vi "Automatische Umschaltung.vi"(6 "Aktion":T1, 8 "error in (no error)":errorcluster caption="Fehler (Eingang, kein Fehler)", 11 "TCP Connection":refnum<k5>) -> (0 "error out":errorcluster caption="Fehler (Ausgang)", 3 "TCP Connection":refnum<k5>)   [LabVIEW 2020, in "ABB-EL3000.lvlib" / "FID.lvlib"]
uses:
  FID.lvlib
  Aktion automatische Umschaltung.ctl
  FID Kalibrierung/Aktion FID Allgemeindaten.ctl
  Modus.ctl
  FID Kalibrierung/FID Kalibrierung.lvlib
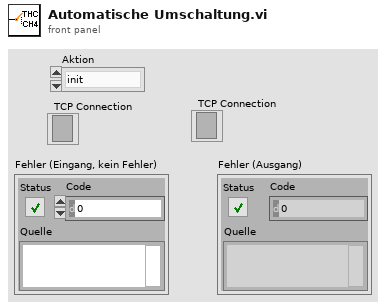
[diagram p1: front panel]
types:
  T1 = typedef "ABB-EL3000.lvlib/FID.lvlib/Aktion automatische Umschaltung.ctl" = enum16{"init", "lesen"}
  T2 = typedef "ABB-EL3000.lvlib/FID.lvlib/Modus.ctl" = enum16{"Automatic", "CH4", "THC", "Efficienty measure", "Switching time"}
  T3 = typedef "ABB-EL3000.lvlib/FID.lvlib/FID Kalibrierung.lvlib/Aktion FID Allgemeindaten.ctl" = enum16{"lesen", "Mod", "Time", "laden", "speichern"}
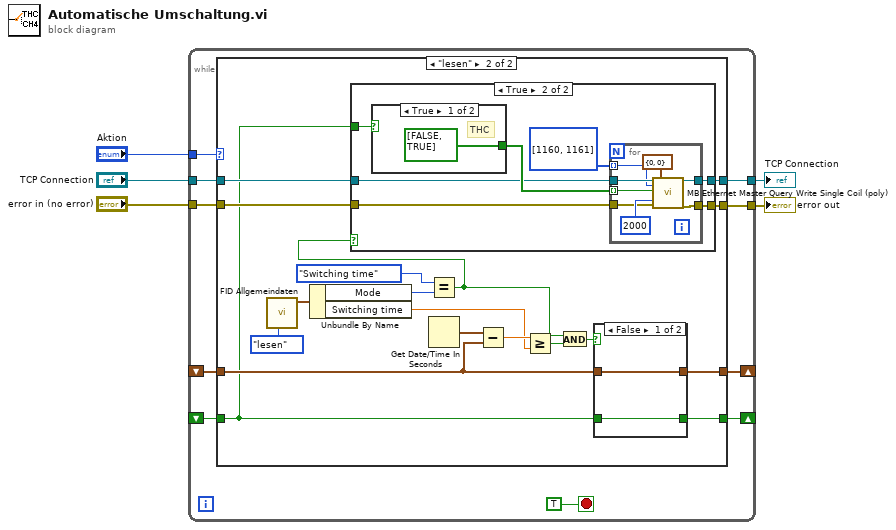
[diagram p0: block diagram]
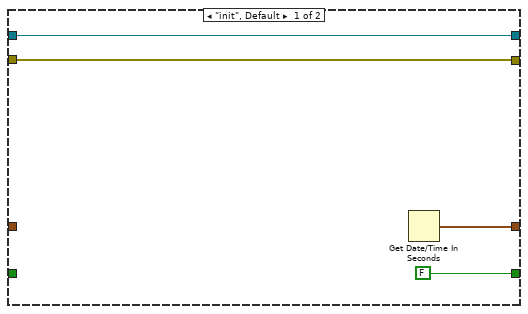
[diagram p2: hidden frame]
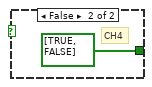
[diagram p4: hidden frame]
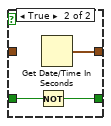
[diagram p5: hidden frame]
diagram:
  n1 = while {
    tunnel: "Aktion" -> [w14]
    shift-right: [w13] -> _
    shift-left: _ -> [w12]
    shift-right: [w11] -> _
    shift-left: _ -> [w10]
    tunnel: "error in (no error)" -> [w7]
    tunnel: "TCP Connection" -> [w9]
    tunnel: [w8] -> w3
    tunnel: [w6] -> w1
    stop <- TRUE stop-if-true
    n2 = case shown="\"lesen\"" w14 {
      tunnel: [w19 w32] -> w13
      tunnel: w12 -> [_ w33]
      tunnel: [FALSE w29] -> w11
      tunnel: w10 -> [_ w24]
      tunnel: w9 -> [w17 w28]
      tunnel: [w17 w27] -> w8
      tunnel: w7 -> [w16 w26]
      tunnel: [w16 w25] -> w6
      frame "init", Default {
        n3 = Get Date/Time In Seconds() -> (seconds since 1Jan1904=w19:timestamp)
      }
      frame "lesen" {
        n4 = call "FID Allgemeindaten.vi"("Aktion"=Aktion_FID_Allgemeindaten."lesen") -> ("FID Allgemein"=w37:cluster{"Mode":T2, "Switching time":sgl})  [unwired: 9 in, 1 out]
        n5 = Unbundle By Name(w37) -> ("Mode"=w21:T2, "Switching time"=w22:sgl)
        n6 = Equal?(x=Modus."Switching time" ("y"), y=w21) -> (x = y?=w23:bool)
        n7 = case shown="True" w23 {
          tunnel: w28 -> [w39 w44]
          tunnel: [w39 w43] -> w27
          tunnel: w26 -> [w38 w42]
          tunnel: [w38 w41] -> w25
          tunnel: w24 -> [_ w40]
          frame False {
          }
          frame True {
            n8 = case shown="True" w40 {
              tunnel: [bool[] [FALSE, TRUE] bool[] [TRUE, FALSE]] -> w46
              frame True {
                # "THC"
              }
              frame False {
                # "CH4"
              }
            }
            n9 = for {
              tunnel: w44 -> [w54]
              tunnel: [w53] -> w43
              tunnel: w42 -> [w52]
              tunnel: [w51] -> w41
              tunnel: u16[] [1160, 1161] -> [w50] mode=indexing
              tunnel: w46 -> [w49] mode=indexing
              n10 = call <userlib>:"MB Ethernet Master Query Write Single Coil (poly).vi"("TCP Connection Refnum in"=w54, "Address"=w50, "Coil"=w49, "Timeout"=u32 2000, "error in"=w52, "MBAP Header"=cluster{"Transaction ID":u16, "Unit ID":u8} {"Transaction ID"=0, "Unit ID"=0}) -> ("TCP Connection Refnum (dup)"=w53:refnum<k5>, "error out"=w51:errorcluster)  [unwired: 11 in, 1 out]
            }
          }
        }
        n11 = Get Date/Time In Seconds() -> (seconds since 1Jan1904=w35:timestamp)
        n12 = Subtract(x=w35, y=w33) -> (x-y=w34:dbl)
        n13 = Greater Or Equal?(x=w34, y=w22) -> (x >= y?=w31:bool)
        n14 = And(x=w23, y=w31) -> (x .and. y?=w30:bool)
        n15 = case shown="False" w30 {
          tunnel: w33 -> [w58 _]
          tunnel: [w58 w61] -> w32
          tunnel: w24 -> [w57 w60]
          tunnel: [w57 w59] -> w29
          frame False {
          }
          frame True {
            n16 = Not(x=w60) -> (.not. x?=w59:bool)
            n17 = Get Date/Time In Seconds() -> (seconds since 1Jan1904=w61:timestamp)
          }
        }
      }
    }
  }
  "TCP Connection" <- w3
  "error out" <- w1
